vi "set_enable_disable_state.vi"(0 "reference (in)":i32, 2 "state (def=OFF)":bool, 5 "error in (no error)":errorcluster) -> (14 "reference (dup)":i32, 17 "success?":bool, 19 "error out":errorcluster)   [LabVIEW 2012]
doc: "This VI is used to enable or disable motor motion control. If disabled, the device can and will receive motion-related commands, but the motor will not respond until it has been enabled.\n\nProduced By:\n\nChristopher Lemieux\nKod Integrations, LLC\n4835 Marianne Drive\nMount Airy, MD 21771\nhttp://www.kodintegrations.com\nemail: clemieux@kodintegrations.com\nphone: (240) 687-1288"
uses:
  main_functions/commands.ctl
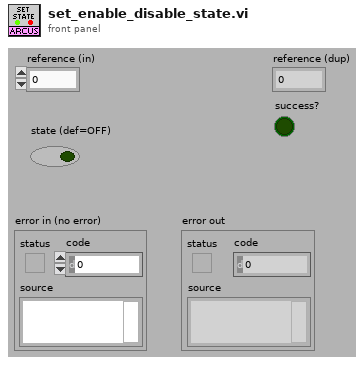
[diagram p1: front panel]
types:
  T1 = typedef "commands.ctl" = enum16{"clear error", "constant jog(-)", "constant jog(+)", "get acceleration", "get actual current", "get device id", "get digital input status", "get digial inputs status", "get dig output status", "get digital outputs status", "get firmware ver", "get high speed", "get idle current", "get low speed", "get micro step", "get motor status", "get move mode", "get polarity", "get position", "get product id", "get power status", "get run current", "get status", "home(-)", "home(+)", "move to position", "power down", "power up", "set acceleration", "set device id", "set digital output", "set digital outputs", "set high speed", "set idle current", "set low speed", "set move mode absolute", "set move mode increment", "set polarity", "set position", "set run current", "stop immediate", "stop slow", "store to memory"}
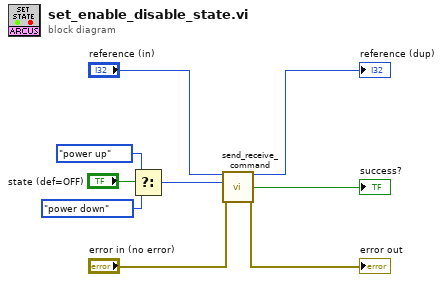
[diagram p0: block diagram]
diagram:
  n1 = Select(t=commands."power up" ("command"), s="state (def=OFF)", f=commands."power down" ("command")) -> (s? t:f=w2:T1)
  n2 = call "send_receive_command.vi"("reference (in)"="reference (in)", "command"=w2, "error in (no error)"="error in (no error)") -> ("reference (dup)"=→"reference (dup)":i32, "success?"=→"success?":bool, "error out"=→"error out":errorcluster)  [unwired: 8 in, 2 out]
